vi "Create.vi"(8 "Error In":errorcluster, 11 "FPGA Reference":T1) -> (0 "Error Out":errorcluster, 3 "Screen Out":refnum<class "Neopixel - Host.lvclass">)   [LabVIEW 2021, in "Neopixel - Host.lvclass"]
uses:
  Neopixel - Host.lvclass
  Controls/FPGA Reference.ctl
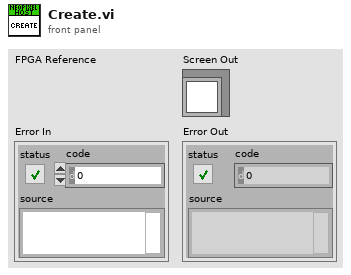
[diagram p1: front panel]
types:
  T1 = typedef "Neopixel - Host.lvclass/FPGA Reference.ctl" = refnum<k20>
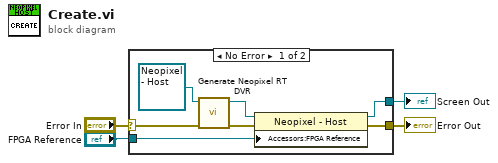
[diagram p0: block diagram]
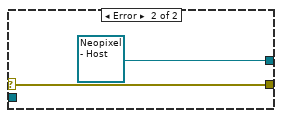
[diagram p2: hidden frame]
diagram:
  n1 = case shown="No Error" "Error In" {
    selector: "Error In" -> [w10 w13]
    tunnel: [w5 w13] -> w3
    tunnel: [w6 refnum<class "Neopixel - Host.lvclass"> refnum ("Screen.lvclass")] -> w2
    tunnel: "FPGA Reference" -> [w7 _]
    frame No Error {
      n2 = call "Generate Neopixel RT DVR.vi"("Error In"=w10, "Display In"=refnum<class "Neopixel - Host.lvclass"> refnum ("Screen.lvclass")) -> ("Error Out"=w8:errorcluster, "Display Out"=w9:refnum<class "Neopixel - Host.lvclass">)  [unwired: 8 in]
      n3 = property class="Neopixel - Host"(reference=w9, error in=w8, "Accessors:FPGA Reference"=w7) -> (reference out=w6:refnum<class "Neopixel - Host.lvclass">, error out=w5:errorcluster)
    }
    frame Error {
    }
  }
  "Screen Out" <- w2
  "Error Out" <- w3
